vi "Create Dot.vi"(7 "3D Stem Property":T4={"General Property"={"Plot Name"="", "Coordinate System"=enum."Cartesian", "Opacity"=0.0}, "Projection Property"={"Draw XY"=FALSE, "Draw YZ"=FALSE, "Draw XZ"=FALSE}, "Plot Property"={"Sprite Type"=enum."Empty Square", "Point Size"=0.0, "Color Ramp Cluster"={"Color Ramp Style"=enum."None", "Color Ramp Array"=[16711934, 393471, 57855, 4390754, 16449346, 16744722, 16711680], "Color Ramp Index"=[45, 91, 133, 175, 219, 255], "Interpolate?"=FALSE, "Logarithm?"=FALSE}, "Line Style"=enum."None", "Line Width"=0.0, "Line Color"=0, "Antialiasing"=FALSE}}, 8 "error in (no error)":errorcluster, 9 "Actual Transform In":T8, 10 "Plot Representation In":T1, 11 "Plot Object In":refnum<vi>) -> (0 "error out":errorcluster, 1 "Actual Transform Out":T8, 2 "Plot Representation Out":T1, 3 "Plot Object Out":refnum<vi>, 4 "Dot Object Out":refnum<vi>)   [LabVIEW 2017, in "3D Stem.lvclass"]
uses:
  <vilib>/Math Plots/3D Math Plots/3D Stem/3D Stem/3D Stem.lvclass
  <vilib>/Math Plots/3D Math Plots/3D Plot/3D Plot/Typedef/Actual Transform.ctl
  <vilib>/Math Plots/3D Math Plots/3D Plot/3D Plot/Typedef/Range Clusters.ctl
  <vilib>/Math Plots/3D Math Plots/3D Plot/3D Plot/Typedef/Plot Representation.ctl
  <vilib>/Math Plots/3D Math Plots/3D Plot/3D Plot/Typedef/Mesh Data.ctl
  <vilib>/Math Plots/3D Math Plots/3D Stem/3D Stem/Typedef/3D Stem Property.ctl
  <vilib>/Math Plots/3D Math Plots/3D Plot/3D Plot/Typedef/Sprite Type.ctl
  <vilib>/Math Plots/3D Math Plots/3D Plot/3D Plot/Typedef/Color Ramp Cluster.ctl
  <vilib>/Math Plots/3D Math Plots/3D Plot/3D Plot/Typedef/Line Type.ctl
  <vilib>/picture/3D Picture Control/Object/Create Object (name).vi
  <vilib>/Math Plots/3D Math Plots/3D Plot/3D Plot/3D Plot.lvclass
  <vilib>/picture/3D Picture Control/NI_3D Picture Control.lvlib
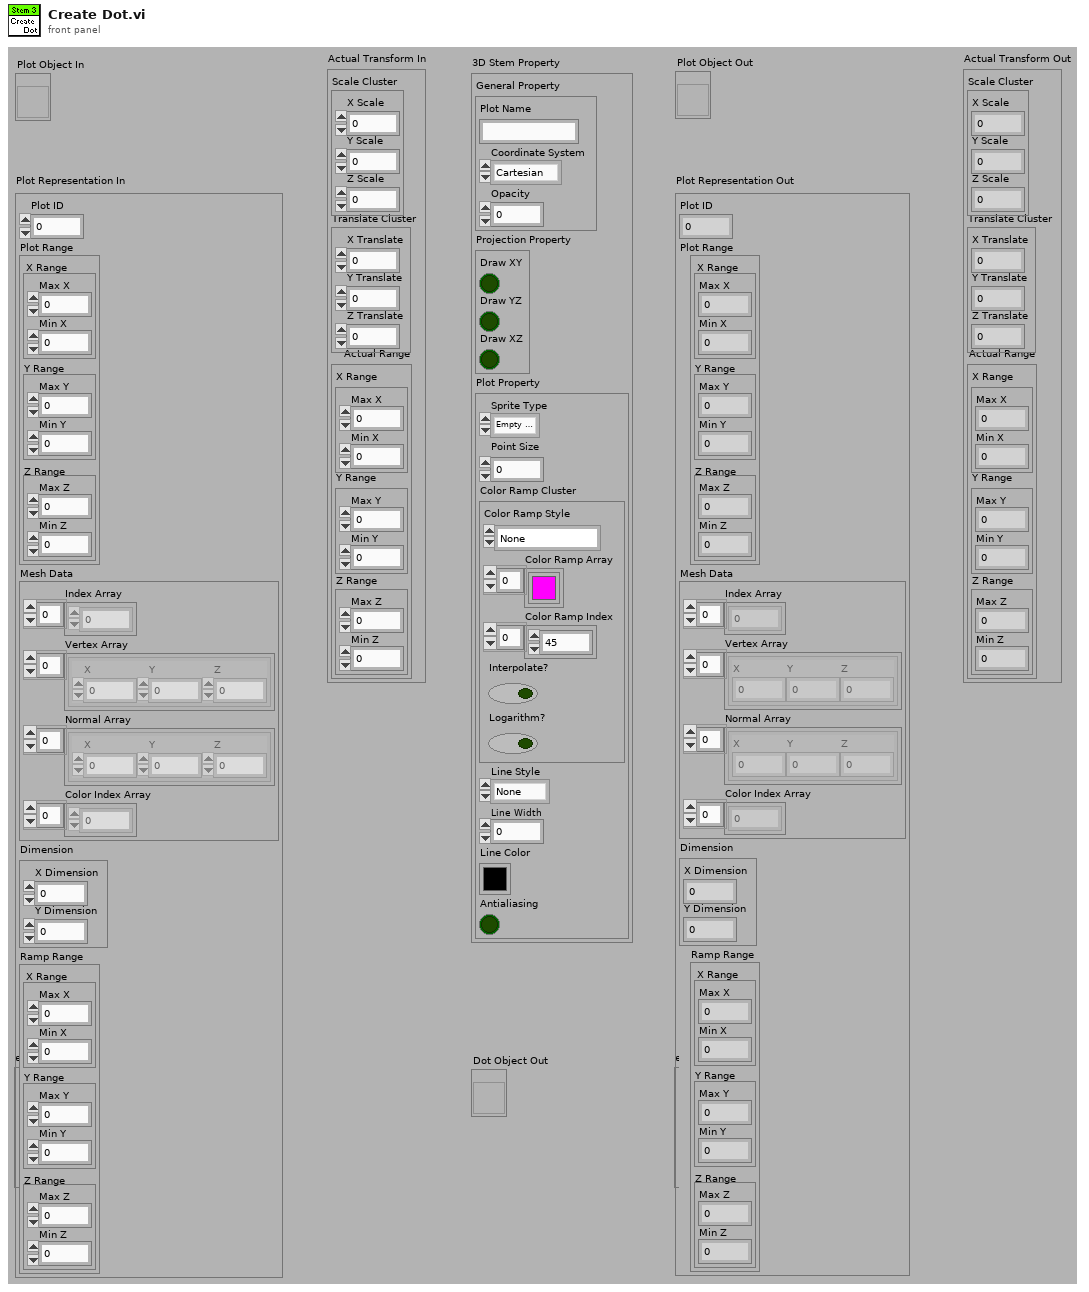
[diagram p1: front panel]
types:
  T1 = typedef "3D Plot.lvclass/Plot Representation.ctl" = cluster{"Plot ID":i32, "Plot Range":T2, "Mesh Data":T3, "Dimension":cluster{"X Dimension":i32, "Y Dimension":i32}, "Ramp Range":T2}
  T2 = typedef "3D Plot.lvclass/Range Clusters.ctl" = cluster{"X Range":cluster{"Max X":sgl, "Min X":sgl}, "Y Range":cluster{"Max Y":sgl, "Min Y":sgl}, "Z Range":cluster{"Max Z":sgl, "Min Z":sgl}}
  T3 = typedef "3D Plot.lvclass/Mesh Data.ctl" = cluster{"Index Array":u32[], "Vertex Array":cluster{"X":sgl, "Y":sgl, "Z":sgl}[], "Normal Array":cluster{"X":sgl, "Y":sgl, "Z":sgl}[], "Color Index Array":i32[]}
  T4 = typedef "3D Stem.lvclass/3D Stem Property.ctl" = cluster{"General Property":cluster{"Plot Name":string, "Coordinate System":enum16{"Cartesian", "Cylindrical", "Spherical"}, "Opacity":sgl}, "Projection Property":cluster{"Draw XY":bool, "Draw YZ":bool, "Draw XZ":bool}, "Plot Property":cluster{"Sprite Type":T5, "Point Size":sgl, "Color Ramp Cluster":T6, "Line Style":T7, "Line Width":sgl, "Line Color":u32, "Antialiasing":bool}}
  T5 = typedef "3D Plot.lvclass/Sprite Type.ctl" = enum16{"None", "Empty Square", "Solid Square", "Empty Diamond", "Solid Diamond", "Empty Circle", "Solid Circle", "Asterisk", "Bold X", "Wireframe Sphere", "Solid Sphere", "Wireframe Cube", "Solid Cube"}
  T6 = typedef "3D Plot.lvclass/Color Ramp Cluster.ctl" = cluster{"Color Ramp Style":enum16{"None", "Shaded", "Color spectrum", "Grey scale", "Custom"}, "Color Ramp Array":u32[], "Color Ramp Index":i32[], "Interpolate?":bool, "Logarithm?":bool}
  T7 = typedef "3D Plot.lvclass/Line Type.ctl" = enum16{"None", "Solid", "Dash", "Dot", "Dash Dot"}
  T8 = typedef "3D Plot.lvclass/Actual Transform.ctl" = cluster{"Scale Cluster":cluster{"X Scale":sgl, "Y Scale":sgl, "Z Scale":sgl}, "Translate Cluster":cluster{"X Translate":sgl, "Y Translate":sgl, "Z Translate":sgl}, "Actual Range":T2}
  T9 = cluster{"X Scale":sgl, "Y Scale":sgl, "Z Scale":sgl}
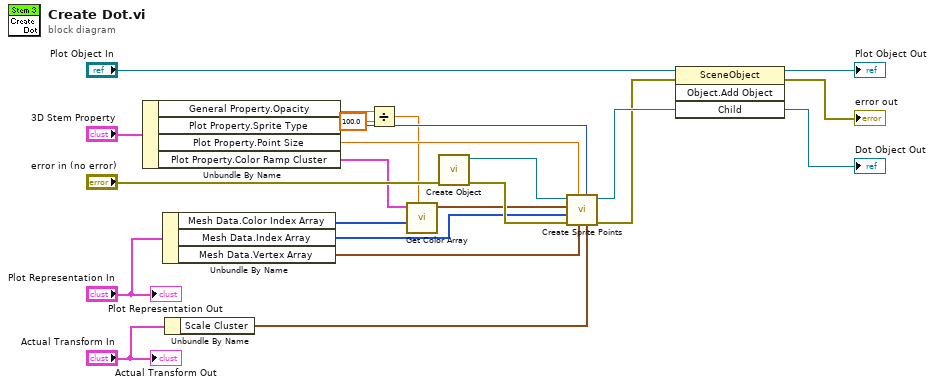
[diagram p0: block diagram]
diagram:
  n1 = Unbundle By Name("3D Stem Property") -> ("General Property.Opacity"=w15:sgl, "Plot Property.Sprite Type"=w12:T5, "Plot Property.Point Size"=w16:sgl, "Plot Property.Color Ramp Cluster"=w5:T6)
  n2 = Unbundle By Name("Plot Representation In") -> ("Mesh Data.Color Index Array"=w7:i32[], "Mesh Data.Index Array"=w3:u32[], "Mesh Data.Vertex Array"=w1:cluster{"X":sgl, "Y":sgl, "Z":sgl}[])
  n3 = Unbundle By Name("Actual Transform In") -> ("Scale Cluster"=w2:T9)
  n4 = Divide(x=w15, y=sgl 100.0) -> (x/y=w6:sgl)
  n5 = call <vilib>:"Get Color Array.vi"("Alpha"=w6, "Color Index Array"=w7, "Color Ramp Cluster"=w5) -> ("Color Array"=w4:cluster{"R":sgl, "G":sgl, "B":sgl, "A":sgl}[])  [unwired: 3 in, 5 out]
  n6 = call-poly <vilib>:"Create Object.vi"("error in (no error)"="error in (no error)") -> ("error out"=w10:errorcluster, "Scene:New Object"=w11:refnum<vi>)  [unwired: 9 in]
  n7 = call <vilib>:"Create Sprite Points.vi"("Scale"=w2, "Sprite Type"=w12, "Vertex Array"=w1, "Point Size"=w16, "error in (no error)"=w10, "Index Array"=w3, "Color Array"=w4, "Dot Object In"=w11) -> ("error out"=w8:errorcluster, "Dot Object Out"=w13:refnum<vi>)  [unwired: 2 out]
  n8 = invoke class="SceneObject" method="Object.Add Object"(reference="Plot Object In", error in=w8, "Child"=w13) -> (reference out=→"Plot Object Out":refnum<vi>, error out=→"error out":errorcluster, "Child"=→"Dot Object Out":refnum<vi>)  [unwired: 1 in, 1 out]
  "Actual Transform Out" <- "Actual Transform In"
  "Plot Representation Out" <- "Plot Representation In"
